vi "Write Pre-amp gain.vi"(8 "error in (no error)":errorcluster, 10 "Pre-amp gain":u8(ring) items=["Gain 1", "Gain 2"], 11 "CCDCamera in":refnum<class "Simulated_CCD_Camera.lvclass">) -> (0 "error out":errorcluster, 3 "CCDCamera out":refnum<class "Simulated_CCD_Camera.lvclass">)   [LabVIEW 2018, in "Simulated_CCD_Camera.lvclass"]
uses:
  Simulated_CCD_Camera.lvclass
  Simulated_CCD_Camera.lvclass/Simulated_CCD_Camera.ctl
  Interface/Interface.lvclass
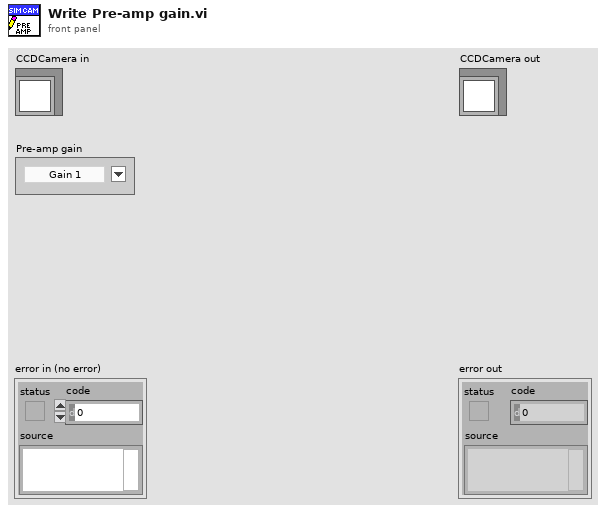
[diagram p1: front panel]
types:
  T1 = cluster{"EXPTIME":sgl, "PREAMP":u8, "READOUT_RATE":u8, "EM_MODE":u8, "EM_GAIN":u16, "BINNING":u16, "INITIAL_LINE":u16, "INITIAL_COLUMN":u16, "FINAL_LINE":u16, "FINAL_COLUMN":u16, "#FRAMES":u32, "SHUTTER_MODE":u8, "COOLER_POWER_STATUS":u16, "TEMP":i8, "#CUBES":u32, "TRIGGER_MODE":u16}
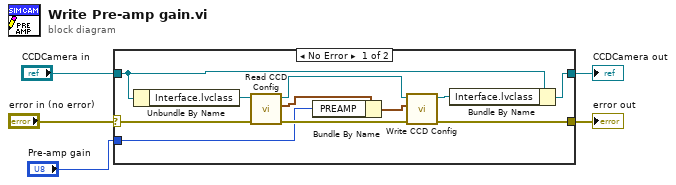
[diagram p0: block diagram]
diagram:
  n1 = case shown="No Error" "error in (no error)" {
    selector: "error in (no error)" -> [w15 w17]
    tunnel: [w14 w17] -> w5
    tunnel: [w13 w18] -> w4
    tunnel: "CCDCamera in" -> [w12 w18]
    tunnel: "Pre-amp gain" -> [w6 _]
    frame No Error {
      n2 = Unbundle By Name(w12) -> ("Interface.lvclass"=w16:refnum<class "Interface.lvclass">)
      n3 = call "Read CCD Config.vi"("error in (no error)"=w15, "Interface in"=w16) -> ("error out"=w9:errorcluster, "CCD Config"=w8:T1, "Interface out"=w10:refnum<class "Interface.lvclass">)  [unwired: 7 in]
      n4 = Bundle By Name(cluster=w8, "PREAMP"=w6) -> (w7:T1)
      n5 = call "Write CCD Config.vi"("error in (no error)"=w9, "CCD Config"=w7, "Interface in"=w10) -> ("error out"=w14:errorcluster, "Interface out"=w11:refnum<class "Interface.lvclass">)  [unwired: 7 in]
      n6 = Bundle By Name(cluster=w12, "Interface.lvclass"=w11) -> (w13:refnum<class "Simulated_CCD_Camera.lvclass">)
    }
    frame Error {
    }
  }
  "error out" <- w5
  "CCDCamera out" <- w4
